vi "Remote Snapshot.vi"() -> ()   [LabVIEW 2010]
panel:
  in  "Snapshot":bool
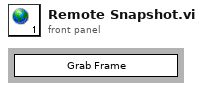
[diagram p1: front panel]
diagram:
